vi "loadTapeParameter.vi"() -> ()   [LabVIEW 2012]
uses:
  <vilib>/addons/database/Connection.llb/DB Tools Open Connec (Path).vi
  <vilib>/addons/database/Connection.llb/Conn Execute.vi
  <vilib>/addons/database/Recordset.llb/Rec Destroy - Connection.vi
  <vilib>/Utility/NIReport.llb/Excel/NI_Excel.lvclass
  <vilib>/Utility/NIReport.llb/NI_report.lvclass
  <vilib>/addons/database/NI_Database_API.lvlib
panel:
  out "error out":errorcluster
  out "output cluster":T1
  in  "Cluster":T1
  out "array 2":string[][](array[string])
  in  "array":string[](array[string])
  out "Vendor":string
  out "row":i32
  in  "template (empty)":path=path "C:/temp/PW-E-25-01E 捲帶包裝封合參數表.xls"
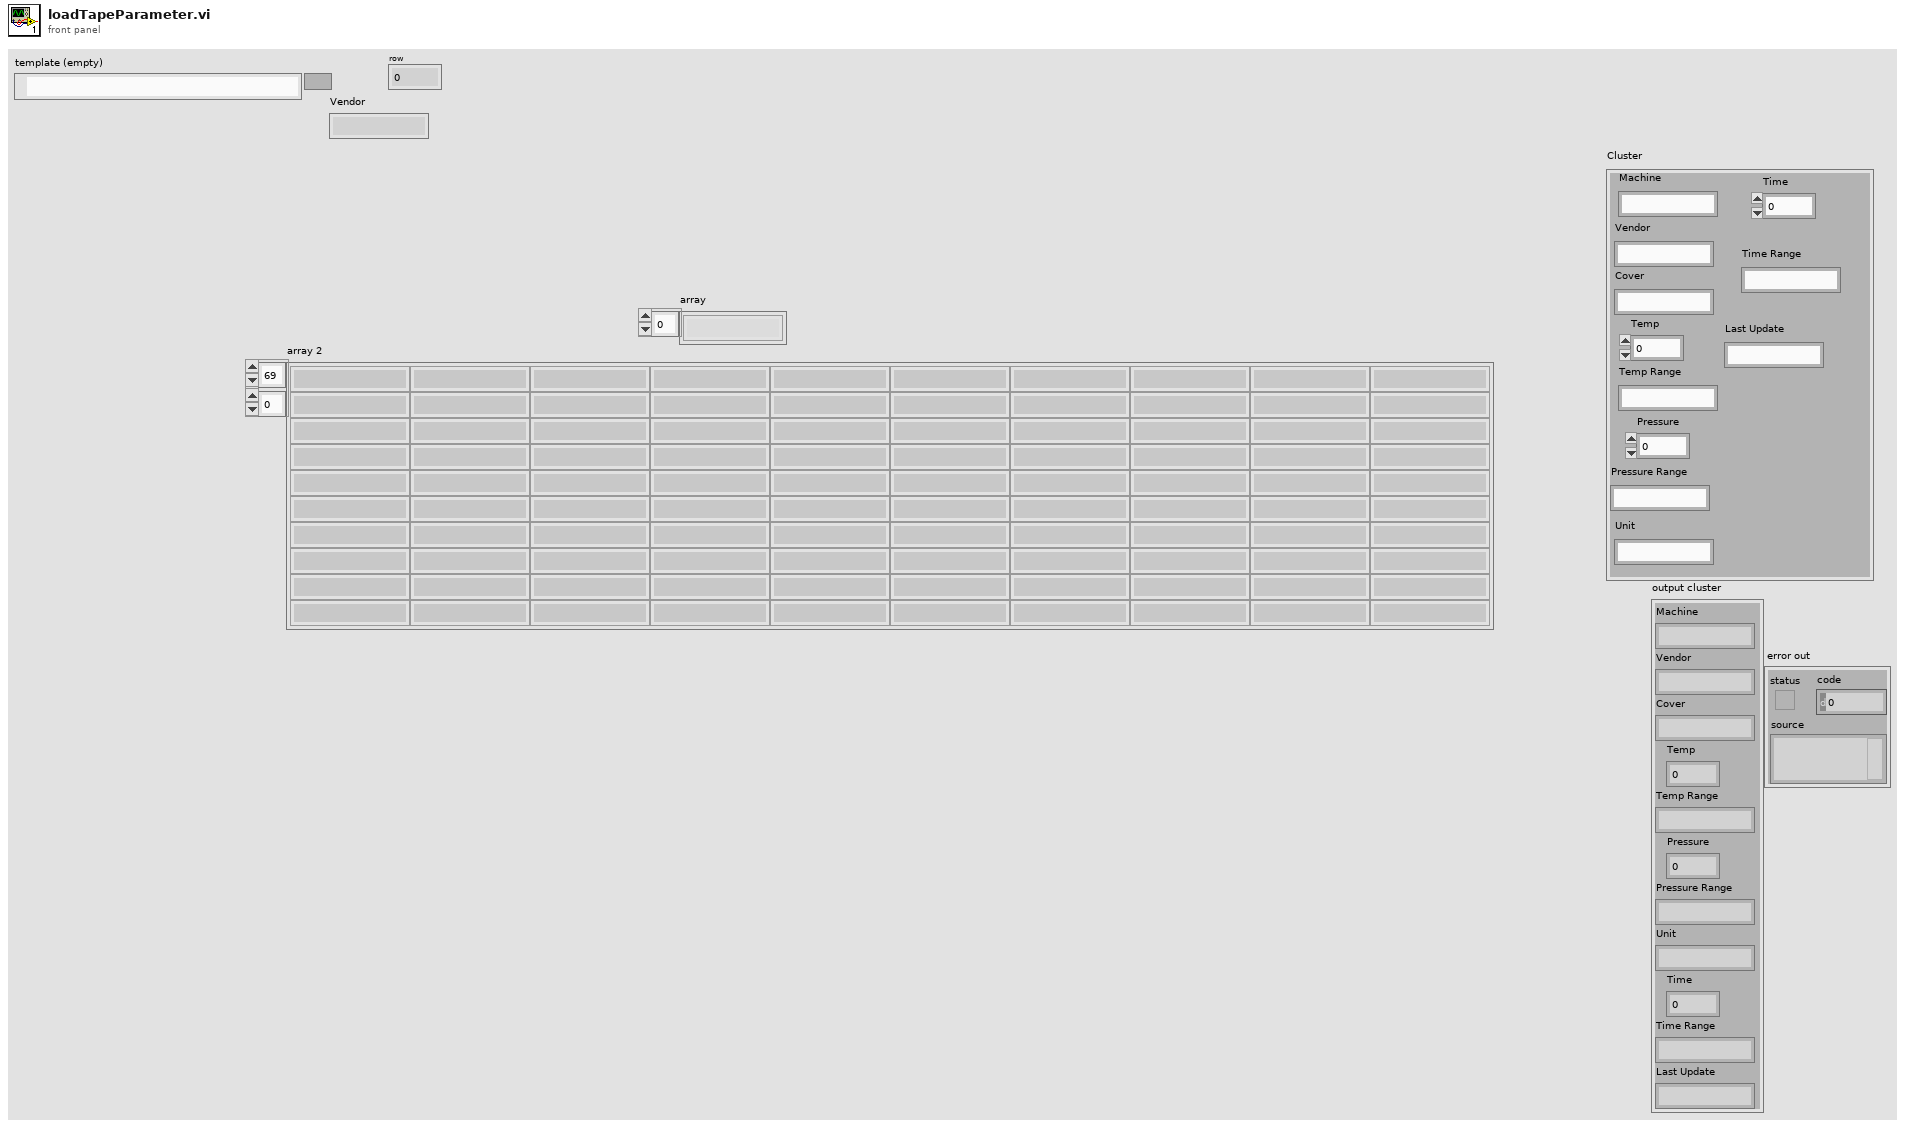
[diagram p1: front panel]
types:
  T1 = cluster{"Machine":string, "Vendor":string, "Cover":string, "Temp":dbl, "Temp Range":string, "Pressure":dbl, "Pressure Range":string, "Unit":string, "Time":dbl, "Time Range":string, "Last Update":string}
  T2 = enum16{"Standard Report", "HTML", "Word", "Excel"}
  T3 = typedef "NI_Database_API.lvlib/Conn ObjectReference.ctl" = refnum<k1>
  T4 = typedef "NI_Database_API.lvlib/Rec ObjectReference.ctl" = refnum<k1>
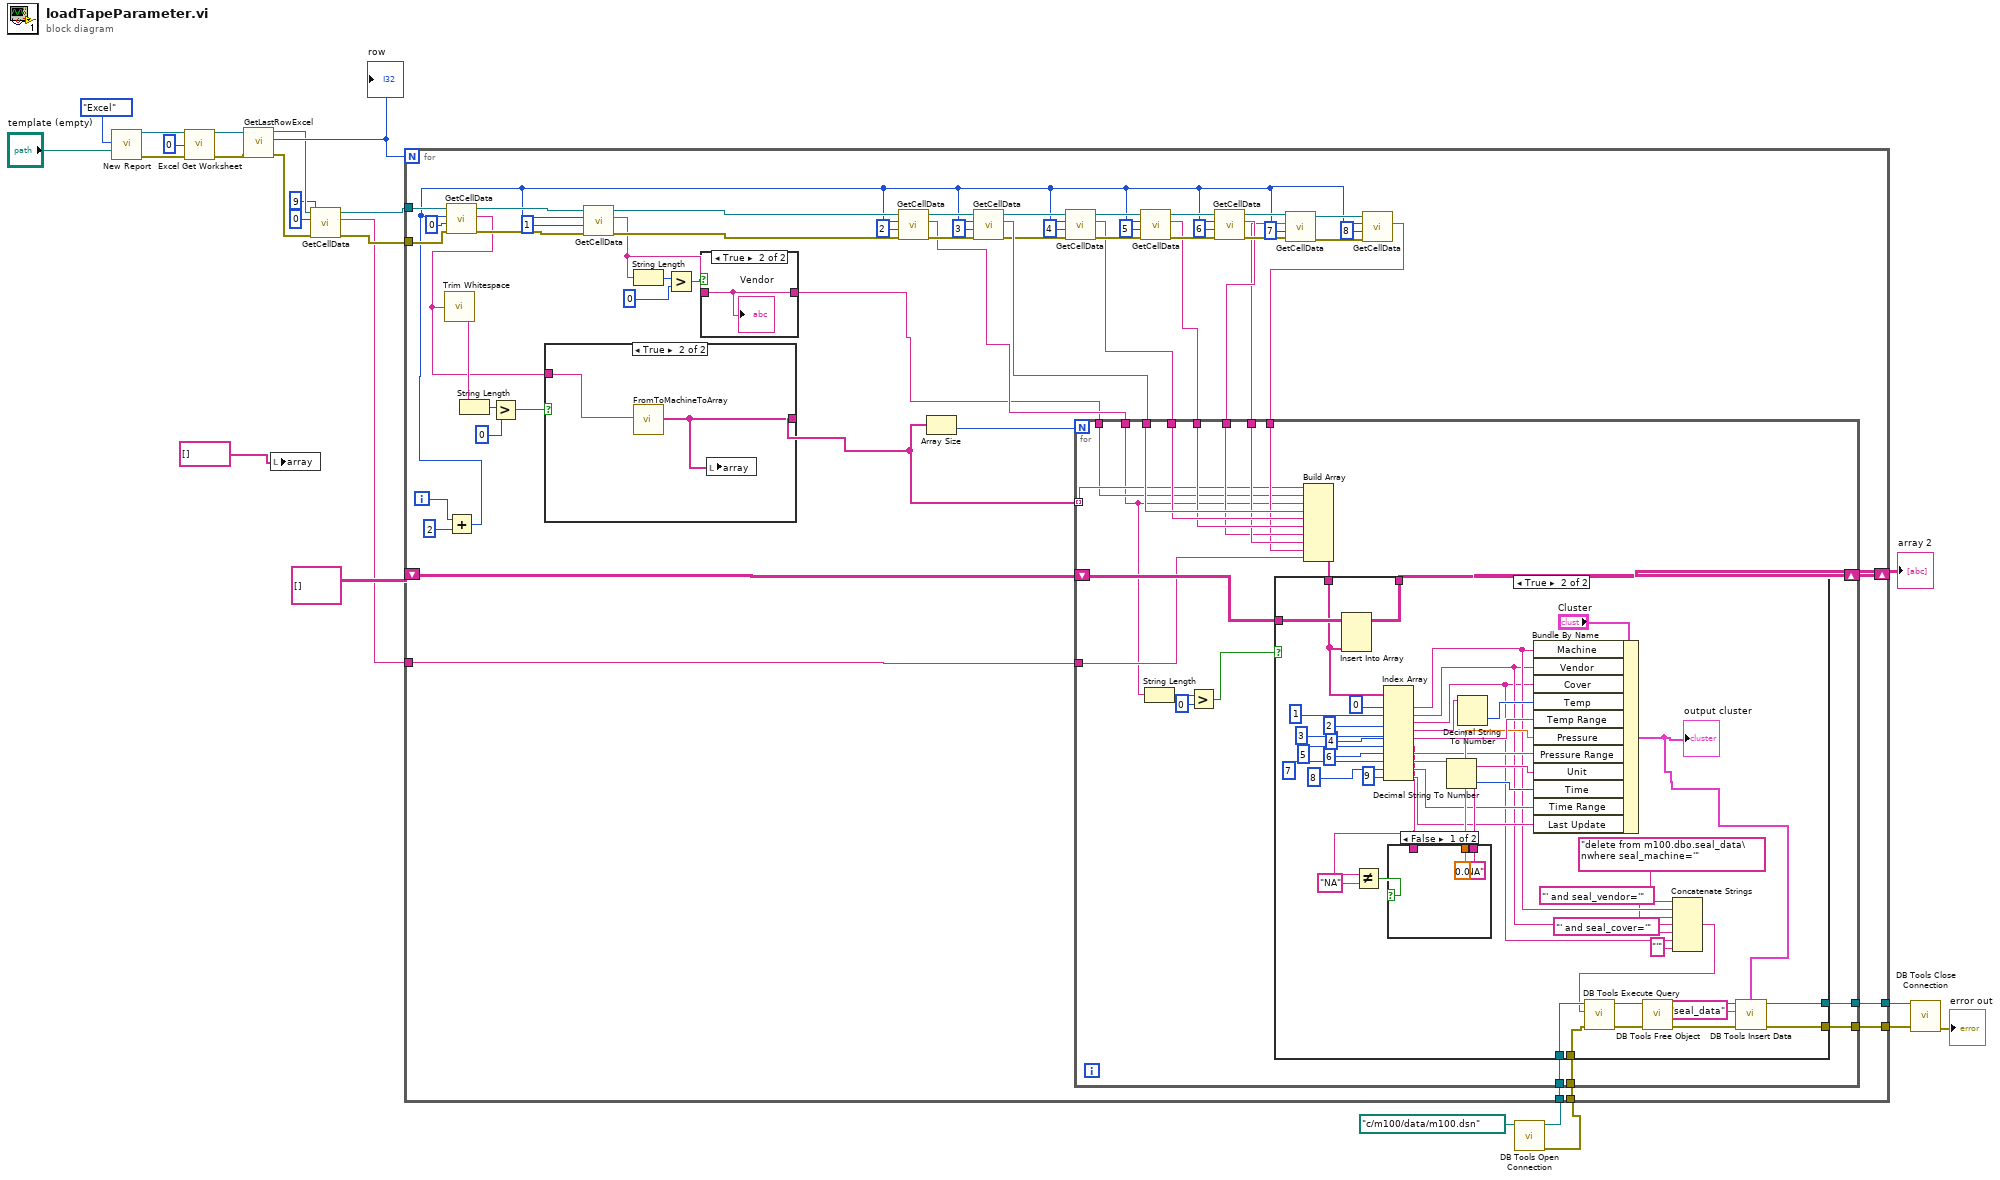
[diagram p0: block diagram]
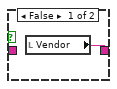
[diagram p2: hidden frame]
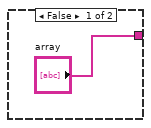
[diagram p3: hidden frame]
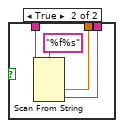
[diagram p5: hidden frame]
diagram:
  n1 = call <vilib>:"New Report.vi"("report type"=T2."Excel" ("Report Type"), "template (empty)"="template (empty)") -> ("report out"=w23:refnum<class "NI_report.lvclass">, "error out"=w22:errorcluster)  [unwired: 12 in]
  n2 = call <vilib>:"Excel Get Worksheet.vi"("report in"=w23, "worksheet index (0)"=0, "error in (no error)"=w22) -> ("report out"=w19:refnum<class "NI_report.lvclass">, "error out"=w18:errorcluster)  [unwired: 11 in]
  n3 = call "GetLastRowExcel.vi"("error in (no error)"=w18, "report in"=w19) -> ("error out"=w10:errorcluster, "row"=w14:i32, "report out"=w11:refnum<class "NI_report.lvclass">)  [unwired: 7 in]
  "row" <- w14
  n4 = local write "array"(string[] [] ("array")) -> ()
  n5 = call "GetCellData.vi"("error in (no error)"=w10, "start column"=9, "start row"=0, "report in"=w11) -> ("error out"=w12:errorcluster, "data"=w7:string, "report out"=w13:refnum<class "NI_report.lvclass">)  [unwired: 5 in]
  n6 = call-poly <vilib>:"DB Tools Open Connection.vi"("connection information"=path "c:/m100/data/m100.dsn") -> ("error out"=w5:errorcluster, "connection reference"=w6:T3)  [unwired: 7 in]
  n7 = for {
    N: w14 -> [_]
    tunnel: w13 -> [w80]
    tunnel: w12 -> [w79]
    shift-right: [w55] -> w15
    shift-left: string[][] [] ("array") -> [w54]
    tunnel: w7 -> [w29]
    tunnel: w6 -> [w28]
    tunnel: w5 -> [w27]
    tunnel: [w26] -> w4
    tunnel: [w25] -> w3
    i -> [w56]
    n8 = Add(x=w56, y=2) -> (x+y=w32:i32)
    n9 = call "GetCellData.vi"("error in (no error)"=w79, "start column"=0, "start row"=w32, "report in"=w80) -> ("error out"=w76:errorcluster, "data"=w62:string, "report out"=w77:refnum<class "NI_report.lvclass">)  [unwired: 5 in]
    n10 = call <vilib>:"Trim Whitespace.vi"("string"=w62) -> ("trimmed string"=w66:string)  [unwired: 1 in]
    n11 = String Length(string=w66) -> (length=w65:i32)
    n12 = Greater?(x=w65, y=0) -> (0:w63:bool)
    n13 = case shown="True" w63 {
      tunnel: w62 -> [_ w85]
      tunnel: ["array" w84] -> w31
      frame False {
      }
      frame True {
        n14 = call "FromToMachineToArray.vi"("string"=w85) -> ("array"=w84:string[])  [unwired: 10 in]
        n15 = local write "array"(w84) -> ()
      }
    }
    n16 = call "GetCellData.vi"("error in (no error)"=w76, "start column"=1, "start row"=w32, "report in"=w77) -> ("error out"=w73:errorcluster, "data"=w58:string, "report out"=w72:refnum<class "NI_report.lvclass">)  [unwired: 5 in]
    n17 = String Length(string=w58) -> (length=w61:i32)
    n18 = Greater?(x=w61, y=0) -> (0:w59:bool)
    n19 = case shown="True" w59 {
      tunnel: w58 -> [_ w82]
      tunnel: [w81 w82] -> w30
      frame False {
        n20 = local read "Vendor"() -> (w81:string)
      }
      frame True {
        "Vendor" <- w82
      }
    }
    n21 = call "GetCellData.vi"("error in (no error)"=w73, "start column"=2, "start row"=w32, "report in"=w72) -> ("error out"=w69:errorcluster, "data"=w33:string, "report out"=w70:refnum<class "NI_report.lvclass">)  [unwired: 5 in]
    n22 = Array Size(array=w31) -> (size(s)=w74:i32)
    n23 = call "GetCellData.vi"("error in (no error)"=w69, "start column"=3, "start row"=w32, "report in"=w70) -> ("error out"=w52:errorcluster, "data"=w67:string, "report out"=w53:refnum<class "NI_report.lvclass">)  [unwired: 5 in]
    n24 = call "GetCellData.vi"("error in (no error)"=w52, "start column"=4, "start row"=w32, "report in"=w53) -> ("error out"=w48:errorcluster, "data"=w38:string, "report out"=w51:refnum<class "NI_report.lvclass">)  [unwired: 5 in]
    n25 = call "GetCellData.vi"("error in (no error)"=w48, "start column"=5, "start row"=w32, "report in"=w51) -> ("error out"=w47:errorcluster, "data"=w37:string, "report out"=w50:refnum<class "NI_report.lvclass">)  [unwired: 5 in]
    n26 = call "GetCellData.vi"("error in (no error)"=w47, "start column"=6, "start row"=w32, "report in"=w50) -> ("error out"=w46:errorcluster, "data"=w36:string, "report out"=w49:refnum<class "NI_report.lvclass">)  [unwired: 5 in]
    n27 = call "GetCellData.vi"("error in (no error)"=w46, "start column"=7, "start row"=w32, "report in"=w49) -> ("error out"=w40:errorcluster, "data"=w35:string, "report out"=w41:refnum<class "NI_report.lvclass">)  [unwired: 5 in]
    n28 = call "GetCellData.vi"("error in (no error)"=w40, "start column"=8, "start row"=w32, "report in"=w41) -> ("data"=w34:string)  [unwired: 5 in, 2 out]
    n29 = for {
      N: w74 -> [_]
      tunnel: w31 -> [w96] mode=indexing
      tunnel: w30 -> [w95]
      tunnel: w67 -> [w105]
      shift-right: [w103] -> w55
      shift-left: w54 -> [w102]
      tunnel: w38 -> [w101]
      tunnel: w37 -> [w100]
      tunnel: w36 -> [w98]
      tunnel: w35 -> [w99]
      tunnel: w34 -> [w97]
      tunnel: w33 -> [w93]
      tunnel: w29 -> [w94]
      tunnel: w28 -> [w89]
      tunnel: w27 -> [w88]
      tunnel: [w87] -> w26
      tunnel: [w86] -> w25
      n30 = String Length(string=w93) -> (length=w92:i32)
      n31 = Greater?(x=w92, y=0) -> (0:w90:bool)
      n32 = Build Array(w96, w95, w93, w105, w101, w100, w98, w99, w97, w94) -> (w104:string[])
      n33 = case shown="True" w90 {
        tunnel: w104 -> [_ w150]
        tunnel: [w108 w153] -> w103
        tunnel: w102 -> [w108 w152]
        tunnel: w89 -> [w107 w126]
        tunnel: w88 -> [w106 w125]
        tunnel: [w107 w111] -> w87
        tunnel: [w106 w110] -> w86
        frame False {
        }
        frame True {
          n34 = Insert Into Array(array=w152, new element=w150) -> (w153:string[][])  [unwired: 2 in]
          n35 = Index Array(array=w150, index #1=0 ("index"), index #2=1 ("index"), index #3=2 ("index"), index #4=3 ("index"), index #5=4 ("index"), index #6=5 ("index"), index #7=6 ("index"), index #8=7 ("index"), index #9=8 ("index"), index #10=9 ("index")) -> (element #1=w121:string, element #2=w119:string, element #3=w117:string, element #4=w139:string, element #5=w137:string, element #6=w129:string, element #7=w134:string, element #8=w133:string, element #9=w131:string, element #10=w130:string)
          n36 = Not Equal?(x=w129, y="NA") -> (x != y?=w127:bool)
          n37 = case shown="False" w127 {
            tunnel: w129 -> [_ w159]
            tunnel: [0.0 w157] -> w136
            tunnel: ["NA" w156] -> w135
            frame False {
            }
            frame True {
              n38 = Scan From String(format string="%f%s", input string=w159) -> (output 1=w157:dbl, output 2=w156:string)  [unwired: 4 in, 3 out]
            }
          }
          n39 = Decimal String To Number(string=w133) -> (number=w132:i32)  [unwired: 2 in, 1 out]
          n40 = Decimal String To Number(string=w139) -> (number=w138:i32)  [unwired: 2 in, 1 out]
          n41 = Bundle By Name(cluster="Cluster", "Machine"=w121, "Vendor"=w119, "Cover"=w117, "Temp"=w138, "Temp Range"=w137, "Pressure"=w136, "Pressure Range"=w134, "Unit"=w135, "Time"=w132, "Time Range"=w131, "Last Update"=w130) -> (w112:T1)
          "output cluster" <- w112
          n42 = Concatenate Strings("delete from m100.dbo.seal_data\nwhere seal_machine='" ("string"), w121, "' and seal_vendor='" ("string"), w119, "' and seal_cover='" ("string"), w117, "'" ("string")) -> (w115:string)
          n43 = call-poly <vilib>:"DB Tools Execute Query.vi"("error in (no error)"=w125, "SQL query"=w115, "connection reference"=w126) -> ("error out"=w122:errorcluster, "recordset reference"=w123:T4)  [unwired: 5 in]
          n44 = call-poly <vilib>:"DB Tools Free Object.vi"("error in (no error)"=w122, "recordset reference"=w123) -> ("error out"=w113:errorcluster, "connection reference"=w114:T3)  [unwired: 8 in]
          n45 = call <vilib>:"DB Tools Insert Data.vi"("data"=w112, "error in (no error)"=w113, "table"="seal_data", "connection reference"=w114) -> ("error out"=w110:errorcluster, "connection reference out"=w111:T3)  [unwired: 6 in]
        }
      }
    }
  }
  "array 2" <- w15
  n46 = call <vilib>:"DB Tools Close Connection.vi"("error in (no error)"=w3, "connection reference"=w4) -> ("error out"=→"error out":errorcluster)  [unwired: 5 in]
